vi "Read Multi Eval Meas Trace EVM Vs Symbol Results.vi"(8 "error in (no error)":errorcluster, 9 "Result Type (Current)":i32(ring) items=["Current"=0, "Average"=1, "Maximum"=4], 10 "Instance (1)":T1=1, 11 "VISA resource name":refnum<visa-resource-name>) -> (0 "error out":errorcluster, 1 "EVM Vs Symbol Results":dbl[](array[numeric]) format="%^.3e", 2 "Reliability":i32, 3 "VISA resource name out":refnum<visa-resource-name>)   [LabVIEW 2015, in "Rohde&Schwarz CMXP NR FR2 Measurement.lvlib"]
doc: "Starts a new single shot measurement and returns the multi eval measurement trace EVM results.\n\nAttributes:\nRSCMXPNRFR2M_ATTR_READ_MULTI_EVAL_MEASUREMENT_TRACE_EVM_VS_SYMBOL_AVERAGE_RESULTS\nRSCMXPNRFR2M_ATTR_READ_MULTI_EVAL_MEASUREMENT_TRACE_EVM_VS_SYMBOL_CURRENT_RESULTS\nRSCMXPNRFR2M_ATTR_READ_MULTI_EVAL_MEASUREMENT_TRACE_EVM_VS_SYMBOL_MAXIMUM_RESULTS\n\nRemote-control commands:\nREAD:NRMMw:MEAS<i>:MEValuation:TRACe:EVMSymbol:AVERage?\nREAD:NRMMw:MEAS<i>:MEValuation:TRACe:EVMSymbol:CURRent?\nREAD:NRMMw:MEAS<i>:MEValuation:TRACe:EVMSymbol:MAXimum?"
uses:
  <instrlib>/Rohde&Schwarz CMXP NR FR2 Measurement/Rohde&Schwarz CMXP NR FR2 Measurement.lvlib
  <instrlib>/Rohde&Schwarz CMXP NR FR2 Measurement/Private/_Instance.ctl
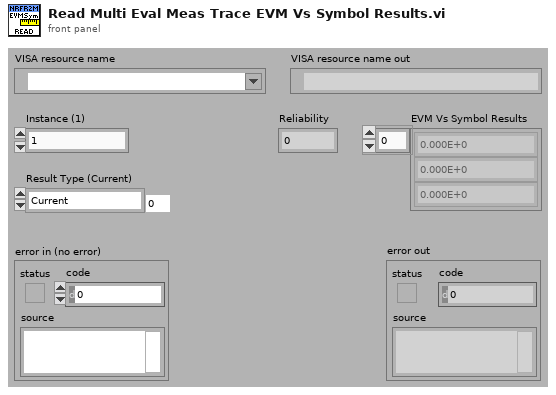
[diagram p1: front panel]
types:
  T1 = typedef "Rohde&Schwarz CMXP NR FR2 Measurement.lvlib/_Instance.ctl" = i32
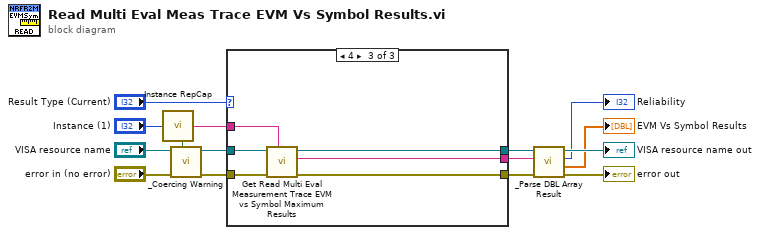
[diagram p0: block diagram]
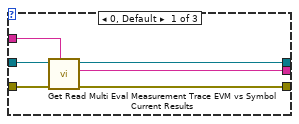
[diagram p2: hidden frame]
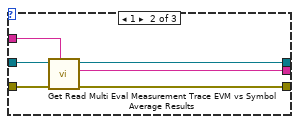
[diagram p3: hidden frame]
diagram:
  n1 = call <instrlib>:"Instance RepCap.vi"("Instance In"="Instance (1)") -> ("In Range?"=w2:bool, "RepCap Identifier Out"=w12:string)  [unwired: 1 in]
  n2 = call <instrlib>:"_Coercing Warning.vi"("In Range?"=w2, "error in (no error)"="error in (no error)", "VISA resource name"="VISA resource name") -> ("error out"=w4:errorcluster, "VISA resource name out"=w3:refnum<visa-resource-name>)  [unwired: 7 in]
  n3 = case shown="4" "Result Type (Current)" {
    tunnel: w4 -> [w21 w27 w33]
    tunnel: w3 -> [w20 w26 w32]
    tunnel: [w19 w25 w31] -> w15
    tunnel: [w18 w24 w30] -> w14
    tunnel: [w17 w23 w29] -> w13
    tunnel: w12 -> [w16 w22 w28]
    frame 0, Default {
      n4 = call "Get Read Multi Eval Measurement Trace EVM vs Symbol Current Results"("Repeated Capabilities"=w16, "error in (no error)"=w21, "instrument handle"=w20) -> ("error out"=w17:errorcluster, "Read Multi Eval Measurement Trace EVM vs Symbol Current Results"=w18:string, "instrument handle out"=w19:refnum<visa-resource-name>)  [unwired: 6 in]
    }
    frame 1 {
      n5 = call "Get Read Multi Eval Measurement Trace EVM vs Symbol Average Results"("Repeated Capabilities"=w22, "error in (no error)"=w27, "instrument handle"=w26) -> ("error out"=w23:errorcluster, "Read Multi Eval Measurement Trace EVM vs Symbol Average Results"=w24:string, "instrument handle out"=w25:refnum<visa-resource-name>)  [unwired: 6 in]
    }
    frame 4 {
      n6 = call "Get Read Multi Eval Measurement Trace EVM vs Symbol Maximum Results"("Repeated Capabilities"=w28, "error in (no error)"=w33, "instrument handle"=w32) -> ("error out"=w29:errorcluster, "Read Multi Eval Measurement Trace EVM vs Symbol Maximum Results"=w30:string, "instrument handle out"=w31:refnum<visa-resource-name>)  [unwired: 6 in]
    }
  }
  n7 = call <instrlib>:"_Parse DBL Array Result.vi"("error in (no error)"=w13, "Input String"=w14, "VISA resource name"=w15) -> ("error out"=→"error out":errorcluster, "Results"=→"EVM Vs Symbol Results":dbl[], "Reliability"=→"Reliability":i32, "VISA resource name out"=→"VISA resource name out":refnum<visa-resource-name>)  [unwired: 5 in]
